vi "Init GPIO.vi"(5 "GPIO Pull (None)":T2, 7 "GPIO Direction":T3, 8 "error in (no error)":errorcluster, 10 "GPIO #":T1=-1, 11 "Session in":refnum<class "Session.lvclass">) -> (0 "error out":errorcluster, 3 "Session out":refnum<class "Session.lvclass">)   [LabVIEW 2024, in "CTI.lvlib" / "Session.lvclass"]
uses:
  Session.lvclass
  GPIO Direction.ctl
  GPIO Pull.ctl
  GPIO Number.ctl
  DeviceComms/DeviceComms.lvclass
  CTI.lvlib
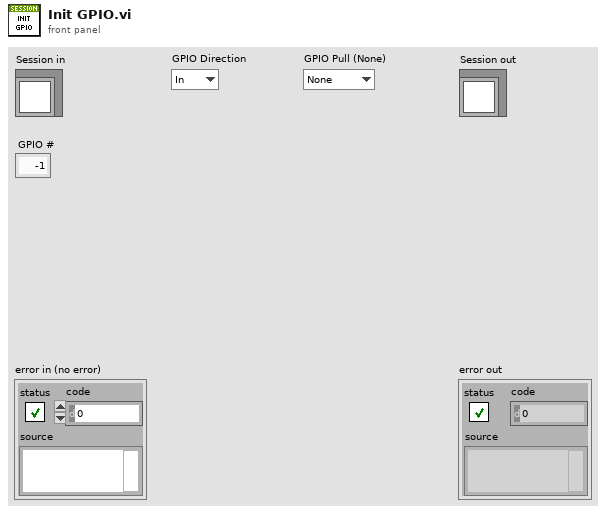
[diagram p1: front panel]
types:
  T1 = typedef "CTI.lvlib/GPIO Number.ctl" = i8
  T2 = typedef "CTI.lvlib/GPIO Pull.ctl" = enum16{"None", "Up", "Down", "Both"}
  T3 = typedef "CTI.lvlib/GPIO Direction.ctl" = enum16{"In", "Out"}
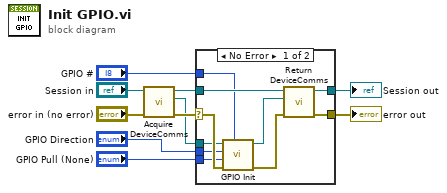
[diagram p0: block diagram]
diagram:
  n1 = call "Acquire DeviceComms.vi"("error in (no error)"="error in (no error)", "Session in"="Session in") -> ("error out"=w10:errorcluster, "DeviceComms"=w7:refnum<class "DeviceComms.lvclass">, "Session out"=w6:refnum<class "Session.lvclass">)  [unwired: 7 in]
  n2 = case shown="No Error" w10 {
    selector: w10 -> [w20 w21]
    tunnel: w7 -> [w19 _]
    tunnel: w6 -> [w18 w22]
    tunnel: "GPIO Direction" -> [w17 _]
    tunnel: "GPIO Pull (None)" -> [w16 _]
    tunnel: "GPIO #" -> [w15 _]
    tunnel: [w14 w22] -> w3
    tunnel: [w11 w21] -> w2
    frame No Error {
      n3 = call-dynamic "GPIO Init.vi"("GPIO #"=w15, "error in (no error)"=w20, "GPIO Pull (None)"=w16, "GPIO Direction"=w17, "DeviceComms in"=w19) -> ("error out"=w12:errorcluster, "DeviceComms out"=w13:refnum<class "DeviceComms.lvclass">)  [unwired: 5 in]
      n4 = call "Return DeviceComms.vi"("error in (no error)"=w12, "DeviceComms"=w13, "Session in"=w18) -> ("error out"=w11:errorcluster, "Session out"=w14:refnum<class "Session.lvclass">)  [unwired: 7 in]
    }
    frame Error {
    }
  }
  "error out" <- w2
  "Session out" <- w3
